vi "Begin.vi"() -> (0 "error out":errorcluster)   [LabVIEW 2011]
doc: "Called before other user functions, this VI is expected to open initial I/O refnums, load in file data, and do all program initialization. Notice that the <B>error out</B> terminal is simply used for data flow. Wiring it to other structures or subVIs ensures that this VI runs first."
uses:
  <vilib>/Rock Robotics/WPI/Joystick/WPI_JoystickDeviceEnum.ctl
  <vilib>/Rock Robotics/SystemInterfaces/DIO/FPGA_DIORelayChannel.ctl
  <vilib>/Rock Robotics/SystemInterfaces/DIO/FPGA_DIOPWMChannel.ctl
  <vilib>/Rock Robotics/SystemInterfaces/DIO/FPGA_DIOChannel.ctl
  <vilib>/Rock Robotics/SystemInterfaces/Typedef/FPGA_TypedefDigitalModule.ctl
  <vilib>/Rock Robotics/WPI/Relay/WPI_RelayDirection.ctl
  <vilib>/Rock Robotics/SystemInterfaces/AI/FPGA_AIGyroChannel.ctl
  <vilib>/Rock Robotics/WPI/Encoder/WPI_EncoderType.ctl
  <vilib>/Rock Robotics/WPI/MotorControl/WPI_MotorControlOpen Victor.vi
  <vilib>/Rock Robotics/WPI/Counter/WPI_CounterDigitalInputToDigitalSource.vi
  Robot Global Data.vi
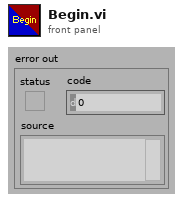
[diagram p1: front panel]
types:
  T1 = typedef "FPGA_AIGyroChannel.ctl" = enum8{"AI 1", "AI 2", "Invalid"}
  T2 = typedef "WPI_EncoderType.ctl" = enum16{"1x", "2x", "4x"}
  T3 = typedef "FPGA_DIOChannel.ctl" = enum8{"DIO 1", "DIO 2", "DIO 3", "DIO 4", "DIO 5", "DIO 6", "DIO 7", "DIO 8", "DIO 9", "DIO 10", "DIO 11", "DIO 12", "DIO 13", "DIO 14", "Invalid"}
  T4 = typedef "FPGA_TypedefDigitalModule.ctl" = enum16{"Digital Module 1", "Digital Module 2"}
  T5 = typedef "WPI_RelayDirection.ctl" = enum16{"Both directions", "Forward only", "Reverse only"}
  T6 = typedef "FPGA_DIOPWMChannel.ctl" = enum8{"PWM 1", "PWM 2", "PWM 3", "PWM 4", "PWM 5", "PWM 6", "PWM 7", "PWM 8", "PWM 9", "PWM 10", "Invalid"}
  T7 = typedef "FPGA_DIORelayChannel.ctl" = enum8{"Relay 1", "Relay 2", "Relay 3", "Relay 4", "Relay 5", "Relay 6", "Relay 7", "Relay 8", "Invalid"}
  T8 = typedef "WPI_JoystickDeviceEnum.ctl" = enum16{"USB 1", "USB 2", "USB 3", "USB 4", "Kinect 1", "Kinect 2"}
  T9 = typedef "WPI_JoystickDevRef.ctl" = cluster{"Device":T8}
  T10 = typedef "WPI_MotorControlDeviceRef.ctl" = cluster{"DeviceStatus":errorcluster, "Type":enum16{"PWM", "CAN"}, "PWM":cluster{"Digital Module":T4, "PWM Channel":T6, "DeadBand":T11}, "CAN":cluster{"Device Number":u8, "Control Mode":T12, "Semaphore":T13, "Max Vout":dbl}, "Invert":bool, "TransformRef":T14, "InvTransformRef":T14}
  T11 = typedef "WPI_PWMDeadband.ctl" = cluster{"Name":string, "maxPositivePwm":i32, "minPositivePwm":i32, "centerPwm":i32, "maxNegativePwm":i32, "minNegativePwm":i32, "angularRange":u16}
  T12 = typedef "WPI_CANJaguar_ControlMode.ctl" = enum8{"Percent VBus", "Current", "Speed", "Position", "Voltage"}
  T13 = typedef "Semaphore RefNum" = refnum<k1>
  T14 = typedef "WPI_PWMTransform_ConPane.ctl" = refnum<vi>
  T15 = typedef "WPI_GyroDevRef.ctl" = cluster{"DevStatus":errorcluster, "Analog Module":T16, "Analog Channel":T17, "Offset":dbl, "Gain (VoltsPerDegree/Second)":dbl}
  T16 = typedef "FPGA_TypedefAnalogModule.ctl" = enum16{"Analog Module 1", "Analog Module 2"}
  T17 = typedef "FPGA_AIChannel.ctl" = enum8{"AI 1", "AI 2", "AI 3", "AI 4", "AI 5", "AI 6", "AI 7", "AI 8", "Invalid"}
  T18 = typedef "WPI_RelayDevRef.ctl" = cluster{"DevStatus":errorcluster, "Relay Channel":T7, "Digital Module":T4, "Relay Direction":T5}
  T19 = typedef "WPI_ServoDeviceRef.ctl" = cluster{"DeviceStatus":errorcluster, "Digital Module":T4, "PWM Channel":T6, "DeadBand":T11}
  T20 = typedef "WPI_DigitalInputDevRef.ctl" = cluster{"DevStatus":errorcluster, "DIO Channel":T3, "Digital Module":T4}
  T21 = typedef "WPI_UltrasonicDeviceRef.ctl" = cluster{"DevStatus":errorcluster, "Ping Digital Module":T4, "Echo Digital Module":T4, "Ping Channel":T3, "Echo Channel":T3, "CntIndex":T22}
  T22 = typedef "FPGA_CounterCtrSystemIndex.ctl" = enum8{"Ctr 0", "Ctr 1", "Ctr 2", "Ctr 3", "Ctr 4", "Ctr 5", "Ctr 6", "Ctr 7", "Invalid"}
  T23 = typedef "FPGA_CounterEncoderSourceConvertionLVSourceType.ctl" = cluster{"DevStatus":errorcluster, "AnalogTriggerMode?":bool, "DigitalMode":cluster{"Digital Module":T4, "DIO Channel":T24}, "AnalogTriggerMode":cluster{"AnalogTriggerIndex":T25, "OutputType":T26}}
  T24 = typedef "FPGA_DIODigitalSourceChannel.ctl" = enum8{"DIO 1", "DIO 2", "DIO 3", "DIO 4", "DIO 5", "DIO 6", "DIO 7", "DIO 8", "DIO 9", "DIO 10", "DIO 11", "DIO 12", "DIO 13", "DIO 14", "Disabled"}
  T25 = typedef "FPGA_AnalogTriggerIndex.ctl" = enum8{"Trig 0", "Trig 1", "Trig 2", "Trig 3", "Trig 4", "Trig 5", "Trig 6", "Trig 7", "Invalid"}
  T26 = typedef "FPGA_AnalogTriggerOutType.ctl" = enum16{"InWindow", "TriggerState", "Rising", "Falling"}
  T27 = typedef "WPI_SerialPortRef.ctl" = cluster{"DevStatus":errorcluster, "Serial Port Name":refnum<visa-resource-name>}
  T28 = typedef "WPI_EncoderDevRef.ctl" = cluster{"DevStatus":errorcluster, "EncoderIndex":T29, "CounterIndex":T22, "DistancePerCount":dbl, "Decoding Type":T2}
  T29 = typedef "FPGA_EncoderIdx.ctl" = enum8{"Enc 0", "Enc 1", "Enc 2", "Enc 3", "Invalid"}
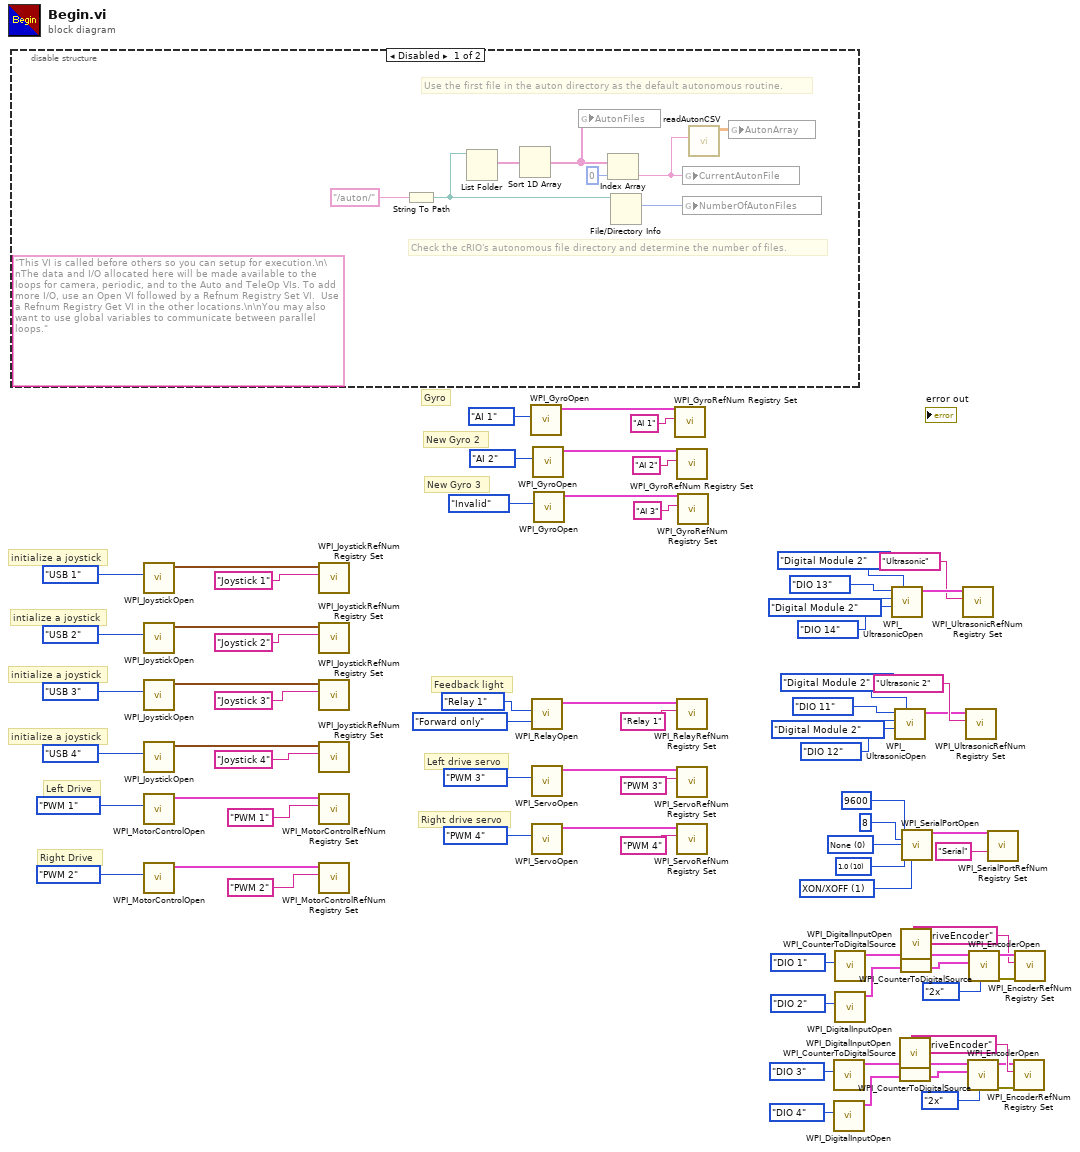
[diagram p0: block diagram]
diagram:
  w43 = u16 10 items=["1.0"=10, "1.5"=15, "2.0"=20] ("Stop Bits")
  w44 = u16 0 items=["None", "Odd", "Even", "Mark", "Space"] ("Parity")
  w47 = u16 1 items=["None", "XON/XOFF", "RTS/CTS", "XON/XOFF & RTS/CTS", "DTR/DSR", "XON/XOFF & DTR/DSR"] ("Flow Control")
  # "New Gyro 3"
  # "New Gyro 2"
  # "Gyro"
  # "Right drive servo"
  # "Left Drive"
  # "Right Drive"
  # "Left drive servo"
  # "Feedback light"
  # "initialize a joystick"
  # "initialize a joystick"
  # "intialize a joystick"
  # "initialize a joystick"
  n1 = disable-structure shown="Disabled" {
    frame Disabled {
      (unwired) "This VI is called before others so you can setup for execution.\n\nThe data and I/O allocated here will be made available to the loops for camera, periodic, and to the Auto and TeleOp VIs. To add more I/O, use an Open VI followed by a Refnum Registry Set VI.  Use a Refnum Registry Get VI in the other locations.\n\nYou may also want to use global variables to communicate between parallel loops."
      # "Check the cRIO's autonomous file directory and determine the number of files."
      # "Use the first file in the auton directory as the default autonomous routine."
      n2 = String To Path(string="/auton/") -> (path=w83:path)
      n3 = List Folder(path=w83) -> (filenames=w82:string[])  [unwired: 1 in, 5 out]
      n4 = Sort 1D Array(array=w82) -> (sorted array=w79:string[])
      n5 = global write "Robot Global Data.vi" "AutonFiles"(w79) -> ()
      n6 = Index Array(array=w79, index=0) -> (element=w77:string)
      n7 = File/Directory Info(path=w83) -> (size=w81:i64)  [unwired: 1 in, 6 out]
      n8 = global write "Robot Global Data.vi" "CurrentAutonFile"(w77) -> ()
      n9 = global write "Robot Global Data.vi" "NumberOfAutonFiles"(w81) -> ()
      n10 = call "readAutonCSV.vi"("AutonFile"=w77) -> ("AutonArray"=w78:dbl[][])  [unwired: 7 out]
      n11 = global write "Robot Global Data.vi" "AutonArray"(w78) -> ()
    }
    frame Enabled {
    }
  }
  n12 = call <vilib>:"WPI_JoystickOpen.vi"("JoystickDevice"=WPI_JoystickDeviceEnum."USB 1") -> ("JoystickDevRef"=w76:T9)  [unwired: 10 out]
  n13 = call <vilib>:"WPI_JoystickOpen.vi"("JoystickDevice"=WPI_JoystickDeviceEnum."USB 2") -> ("JoystickDevRef"=w71:T9)  [unwired: 10 out]
  n14 = call <vilib>:"WPI_JoystickOpen.vi"("JoystickDevice"=WPI_JoystickDeviceEnum."USB 3") -> ("JoystickDevRef"=w70:T9)  [unwired: 10 out]
  n15 = call <vilib>:"WPI_JoystickOpen.vi"("JoystickDevice"=WPI_JoystickDeviceEnum."USB 4") -> ("JoystickDevRef"=w65:T9)  [unwired: 10 out]
  n16 = call-poly <vilib>:"WPI_MotorControlOpen.vi"("PWM Channel"=FPGA_DIOPWMChannel."PWM 1") -> ("MotorControlDeviceRef"=w55:T10)  [unwired: 6 in, 4 out]
  n17 = call-poly <vilib>:"WPI_MotorControlOpen.vi"("PWM Channel"=FPGA_DIOPWMChannel."PWM 2") -> ("MotorControlDeviceRef"=w56:T10)  [unwired: 6 in, 4 out]
  n18 = call <vilib>:"WPI_JoystickRefNum Registry Set.vi"("refnum name"="Joystick 1", "JoystickDevRef"=w76) -> ()  [unwired: 1 in, 9 out]
  n19 = call <vilib>:"WPI_JoystickRefNum Registry Set.vi"("refnum name"="Joystick 2", "JoystickDevRef"=w71) -> ()  [unwired: 1 in, 9 out]
  n20 = call <vilib>:"WPI_JoystickRefNum Registry Set.vi"("refnum name"="Joystick 3", "JoystickDevRef"=w70) -> ()  [unwired: 1 in, 9 out]
  n21 = call <vilib>:"WPI_JoystickRefNum Registry Set.vi"("refnum name"="Joystick 4", "JoystickDevRef"=w65) -> ()  [unwired: 1 in, 9 out]
  n22 = call <vilib>:"WPI_MotorControlRefNum Registry Set.vi"("refnum name"="PWM 1", "MotorControlDevRef"=w55) -> ()  [unwired: 1 in, 9 out]
  n23 = call <vilib>:"WPI_MotorControlRefNum Registry Set.vi"("refnum name"="PWM 2", "MotorControlDevRef"=w56) -> ()  [unwired: 1 in, 9 out]
  n24 = call <vilib>:"WPI_GyroOpen.vi"("Analog Channel"=FPGA_AIGyroChannel."AI 1") -> ("GyroDevRef"=w35:T15)  [unwired: 5 in, 5 out]
  n25 = call <vilib>:"WPI_RelayOpen.vi"("Relay Direction"=WPI_RelayDirection."Forward only", "Relay Channel"=FPGA_DIORelayChannel."Relay 1") -> ("RelayDevRef"=w64:T18)  [unwired: 2 in, 7 out]
  n26 = call <vilib>:"WPI_ServoOpen.vi"("PWM Channel"=FPGA_DIOPWMChannel."PWM 3") -> ("ServoDeviceRef"=w61:T19)  [unwired: 3 in, 7 out]
  n27 = call <vilib>:"WPI_ServoOpen.vi"("PWM Channel"=FPGA_DIOPWMChannel."PWM 4") -> ("ServoDeviceRef"=w50:T19)  [unwired: 3 in, 7 out]
  n28 = call <vilib>:"WPI_GyroOpen.vi"("Analog Channel"=FPGA_AIGyroChannel."AI 2") -> ("GyroDevRef"=w5:T15)  [unwired: 5 in, 5 out]
  n29 = call <vilib>:"WPI_GyroOpen.vi"("Analog Channel"=FPGA_AIGyroChannel."Invalid") -> ("GyroDevRef"=w4:T15)  [unwired: 5 in, 5 out]
  n30 = call <vilib>:"WPI_GyroRefNum Registry Set.vi"("refnum name"="AI 1", "GyroDevRef"=w35) -> ()  [unwired: 1 in, 9 out]
  n31 = call <vilib>:"WPI_GyroRefNum Registry Set.vi"("refnum name"="AI 2", "GyroDevRef"=w5) -> ()  [unwired: 1 in, 9 out]
  n32 = call <vilib>:"WPI_RelayRefNum Registry Set.vi"("refnum name"="Relay 1", "RelayDevRef"=w64) -> ()  [unwired: 1 in, 9 out]
  n33 = call <vilib>:"WPI_ServoRefNum Registry Set.vi"("refnum name"="PWM 3", "ServoDeviceRef"=w61) -> ()  [unwired: 1 in, 9 out]
  n34 = call <vilib>:"WPI_ServoRefNum Registry Set.vi"("refnum name"="PWM 4", "ServoDeviceRef"=w50) -> ()  [unwired: 1 in, 9 out]
  n35 = call <vilib>:"WPI_GyroRefNum Registry Set.vi"("refnum name"="AI 3", "GyroDevRef"=w4) -> ()  [unwired: 1 in, 9 out]
  n36 = call <vilib>:"WPI_DigitalInputOpen.vi"("DIO Channel"=FPGA_DIOChannel."DIO 3") -> ("DigitalInputDevRef"=w9:T20)  [unwired: 2 in, 8 out]
  n37 = call <vilib>:"WPI_DigitalInputOpen.vi"("DIO Channel"=FPGA_DIOChannel."DIO 4") -> ("DigitalInputDevRef"=w10:T20)  [unwired: 2 in, 8 out]
  n38 = call <vilib>:"WPI_DigitalInputOpen.vi"("DIO Channel"=FPGA_DIOChannel."DIO 1") -> ("DigitalInputDevRef"=w24:T20)  [unwired: 2 in, 8 out]
  n39 = call <vilib>:"WPI_DigitalInputOpen.vi"("DIO Channel"=FPGA_DIOChannel."DIO 2") -> ("DigitalInputDevRef"=w23:T20)  [unwired: 2 in, 8 out]
  n40 = call <vilib>:"WPI_UltrasonicOpen.vi"("Ping Digital Module (Module 1)"=FPGA_TypedefDigitalModule."Digital Module 2" ("Ping DIO Module"), "Echo DIO Channel"=FPGA_DIOChannel."DIO 14", "Echo Digital Module (Module 1)"=FPGA_TypedefDigitalModule."Digital Module 2" ("Echo DIO Module"), "Ping DIO Channel"=FPGA_DIOChannel."DIO 13") -> ("UltrasonicDevRef"=w40:T21)  [unwired: 1 in, 6 out]
  n41 = call <vilib>:"WPI_UltrasonicOpen.vi"("Ping Digital Module (Module 1)"=FPGA_TypedefDigitalModule."Digital Module 2" ("Ping DIO Module"), "Echo DIO Channel"=FPGA_DIOChannel."DIO 12", "Echo Digital Module (Module 1)"=FPGA_TypedefDigitalModule."Digital Module 2" ("Echo DIO Module"), "Ping DIO Channel"=FPGA_DIOChannel."DIO 11") -> ("UltrasonicDevRef"=w29:T21)  [unwired: 1 in, 6 out]
  n42 = call-poly <vilib>:"WPI_CounterToDigitalSource.vi"("DigitalInputDevRef"=w9) -> ("Digital Source"=w11:T23)  [unwired: 1 in, 5 out]
  n43 = call-poly <vilib>:"WPI_CounterToDigitalSource.vi"("DigitalInputDevRef"=w10) -> ("Digital Source"=w12:T23)  [unwired: 6 out]
  n44 = call-poly <vilib>:"WPI_CounterToDigitalSource.vi"("DigitalInputDevRef"=w24) -> ("Digital Source"=w22:T23)  [unwired: 1 in, 5 out]
  n45 = call-poly <vilib>:"WPI_CounterToDigitalSource.vi"("DigitalInputDevRef"=w23) -> ("Digital Source"=w21:T23)  [unwired: 6 out]
  n46 = call <vilib>:"WPI_SerialPortOpen.vi"("Baud Rate"=u32 9600, "Data Bits"=u16 8, "Parity"=w44, "Stop Bits"=w43, "Flow Control"=w47) -> ("SerialPortRef"=w49:T27)  [unwired: 4 in, 6 out]
  n47 = call <vilib>:"WPI_UltrasonicRefNum Registry Set.vi"("refnum name"="Ultrasonic", "UltrasonicDevRef"=w40) -> ()  [unwired: 1 in, 9 out]
  n48 = call <vilib>:"WPI_UltrasonicRefNum Registry Set.vi"("refnum name"="Ultrasonic 2", "UltrasonicDevRef"=w29) -> ()  [unwired: 1 in, 9 out]
  n49 = call <vilib>:"WPI_EncoderOpen.vi"("Decoding Type"=WPI_EncoderType."2x", "BSource"=w12, "ASource"=w11) -> ("error out"=w14:errorcluster, "EncoderDevRef"=w13:T28)  [unwired: 5 in, 2 out]
  n50 = call <vilib>:"WPI_EncoderOpen.vi"("Decoding Type"=WPI_EncoderType."2x", "BSource"=w21, "ASource"=w22) -> ("error out"=w19:errorcluster, "EncoderDevRef"=w20:T28)  [unwired: 5 in, 2 out]
  n51 = call <vilib>:"WPI_SerialPortRefNum Registry Set.vi"("refnum name"="Serial", "SerialPortRef"=w49) -> ()  [unwired: 1 in, 9 out]
  n52 = call <vilib>:"WPI_EncoderRefNum Registry Set.vi"("error in (no error)"=w14, "refnum name"="RDriveEncoder", "EncoderDevRef"=w13) -> ()  [unwired: 9 out]
  n53 = call <vilib>:"WPI_EncoderRefNum Registry Set.vi"("error in (no error)"=w19, "refnum name"="LDriveEncoder", "EncoderDevRef"=w20) -> ()  [unwired: 9 out]
